vi "filePathManager.vi"(8 "Error In":errorcluster, 11 "First Call?":bool) -> (0 "Error Out":errorcluster, 2 "info File Path":path, 3 "src File Path":path)   [LabVIEW 2018]
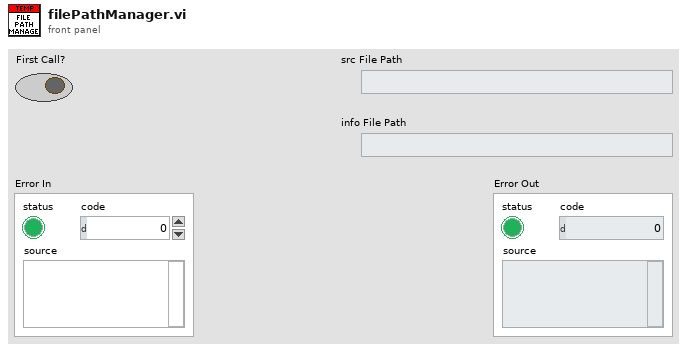
[diagram p1: front panel]
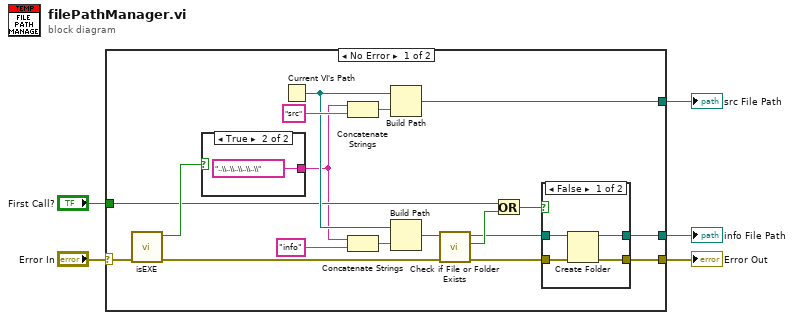
[diagram p0: block diagram]
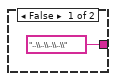
[diagram p3: hidden frame]
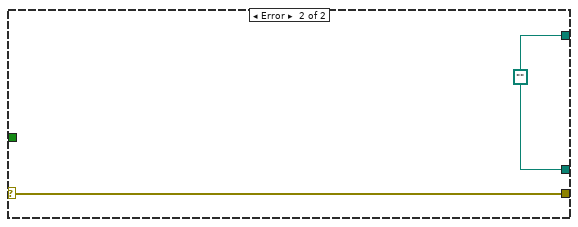
[diagram p4: hidden frame]
diagram:
  n1 = case shown="No Error" "Error In" {
    selector: "Error In" -> [w23 w33]
    tunnel: [w16 w33] -> w4
    tunnel: "First Call?" -> [w13 _]
    tunnel: [w8 w32] -> w2
    tunnel: [w7 w32] -> w1
    frame No Error {
      n2 = call "isEXE.vi"("Error In"=w23) -> ("Error Out"=w14:errorcluster, "isEXE?"=w22:bool)  [unwired: 9 in]
      n3 = case shown="True" w22 {
        tunnel: ["..\\..\\..\\..\\" "..\\..\\..\\..\\..\\"] -> w6
        frame False {
        }
        frame True {
        }
      }
      n4 = Current VI's Path() -> (path=w17:path)
      n5 = Concatenate Strings(w6, "src" ("string")) -> (w21:string)
      n6 = Concatenate Strings(w6, "info" ("string")) -> (w18:string)
      n7 = Build Path(base path=w17, name or relative path=w21) -> (appended path=w8:path)
      n8 = Build Path(base path=w17, name or relative path=w18) -> (appended path=w15:path)
      n9 = call <vilib>:"Check if File or Folder Exists.vi"("error in (no error)"=w14, "path"=w15) -> ("error out"=w10:errorcluster, "file or folder exists?"=w12:bool, "dup path"=w9:path)  [unwired: 7 in]
      n10 = Or(x=w13, y=w12) -> (x .or. y?=w11:bool)
      n11 = case shown="False" w11 {
        tunnel: [w26 w29] -> w16
        tunnel: w10 -> [w27 w29]
        tunnel: w9 -> [w25 w28]
        tunnel: [w24 w28] -> w7
        frame False {
          n12 = Create Folder(path (use dialog)=w25, error in=w27) -> (created path=w24:path, error out=w26:errorcluster)  [unwired: 1 in, 1 out]
        }
        frame True {
        }
      }
    }
    frame Error {
      w32 = path ""
    }
  }
  "Error Out" <- w4
  "src File Path" <- w2
  "info File Path" <- w1
